vi "Parameters_Get_VelocityMove.vi"(11 "Parameters":dbl[](array[numeric])) -> (1 "Acceleration Jerk":dbl=1000.0, 2 "Acceleration":dbl=10000.0, 3 "Velocity":dbl=1000.0)   [LabVIEW 2017, in "WordManipulationLibrary.lvlib"]
uses:
  WordManipulationLibrary.lvlib
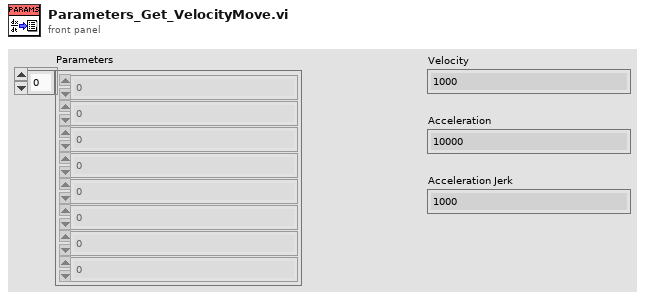
[diagram p1: front panel]
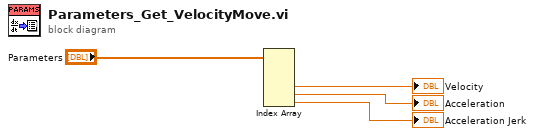
[diagram p0: block diagram]
diagram:
  n1 = Index Array(array="Parameters") -> (element #3=→"Velocity":dbl, element #4=→"Acceleration":dbl, element #5=→"Acceleration Jerk":dbl)  [unwired: 5 in, 2 out]
